vi "Get spectra Freq.vi"() -> (5 "Plug in titles":string[](array[string]), 7 "Plug in values":string[](array[string]))   [LabVIEW 2021]
uses:
  Globals/Meas_global.vi
panel:
  in  "Channel Indices for Spectra":i32[](array[numeric])=[0]
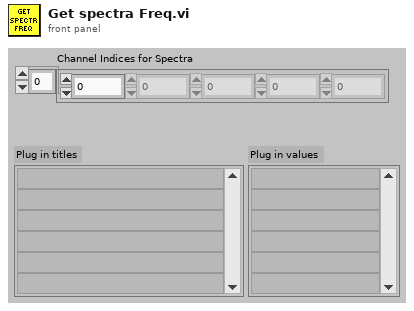
[diagram p1: front panel]
types:
  T1 = typedef "Setup.ctl" = enum16{"Run Program", "Show Setup", "Save Current Setup", "Setup Front Panel"}
  T2 = typedef "XY_Plot_Cluster.ctl" = cluster{"First Name":string, "Second Name":string, "X axis name":string, "Y axis name":string, "X array":dbl[], "Y array":dbl[], "Weighting":dbl[]}
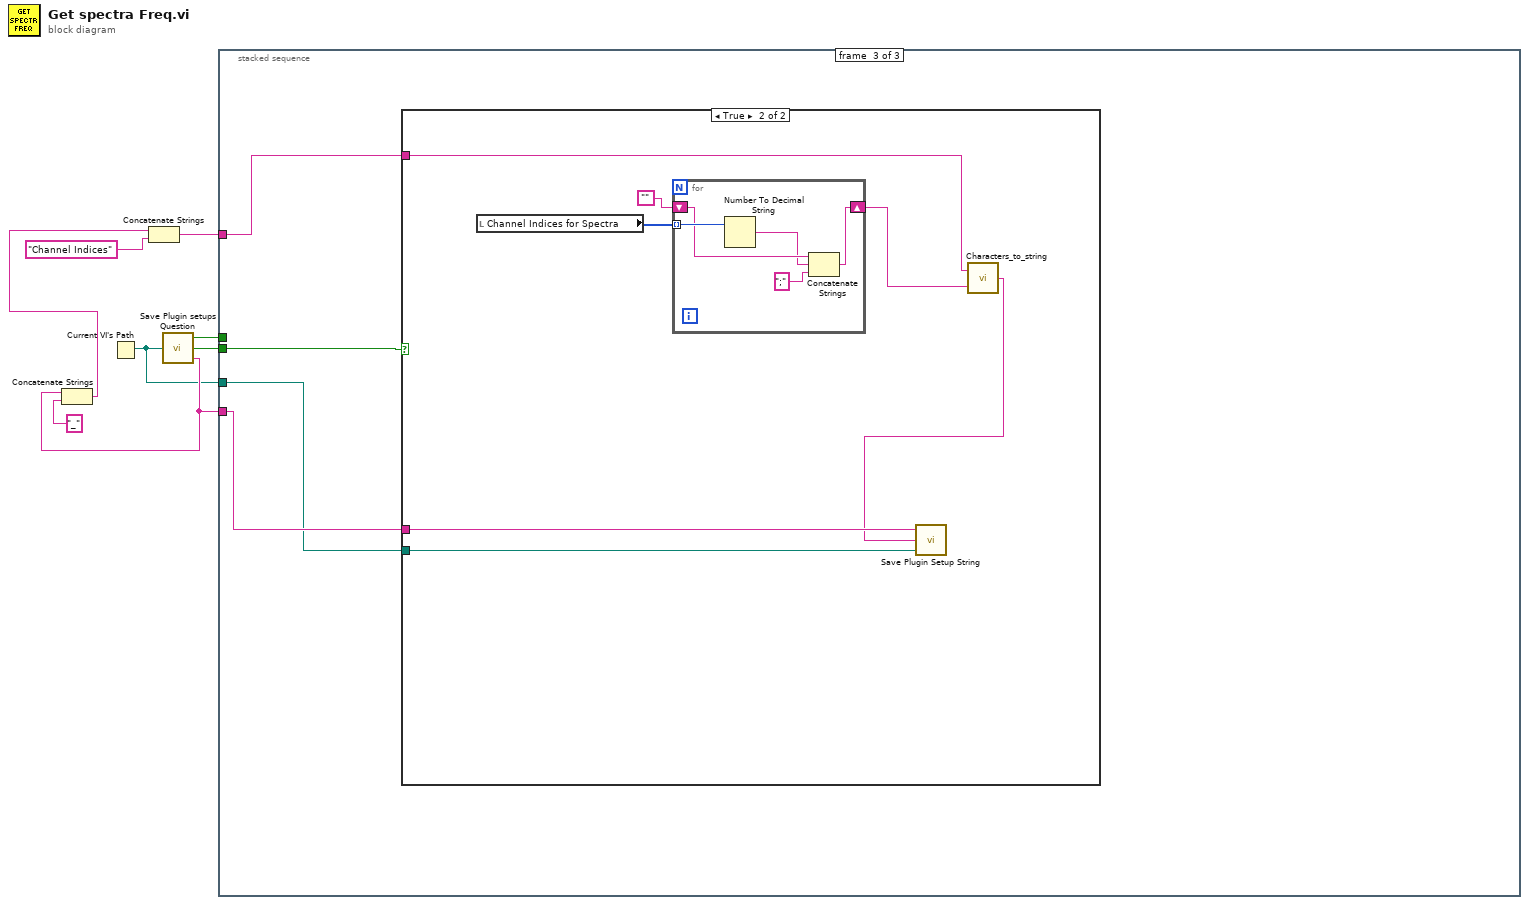
[diagram p0: block diagram]
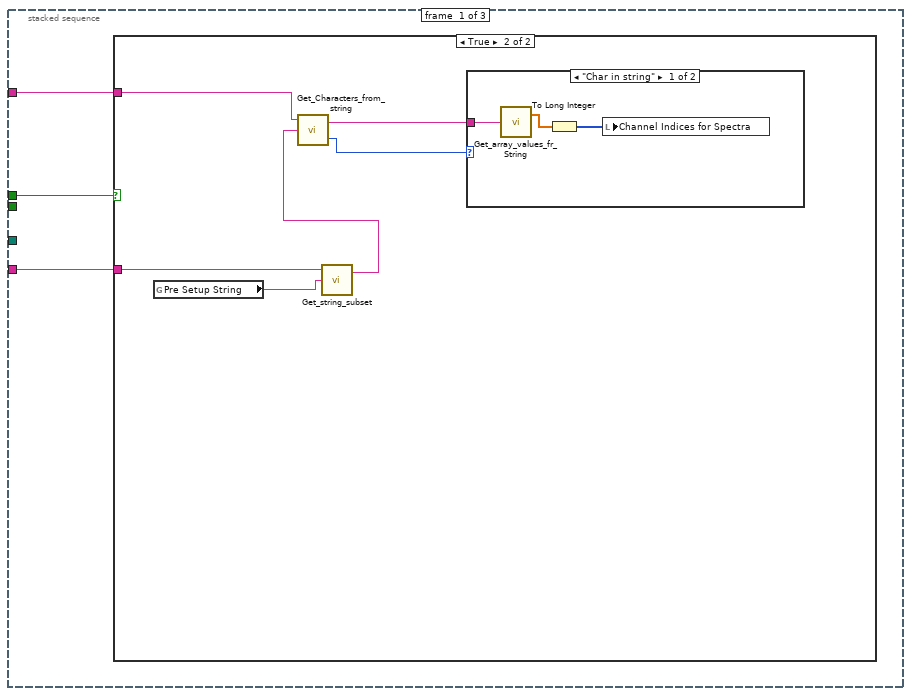
[diagram p2: hidden frame]
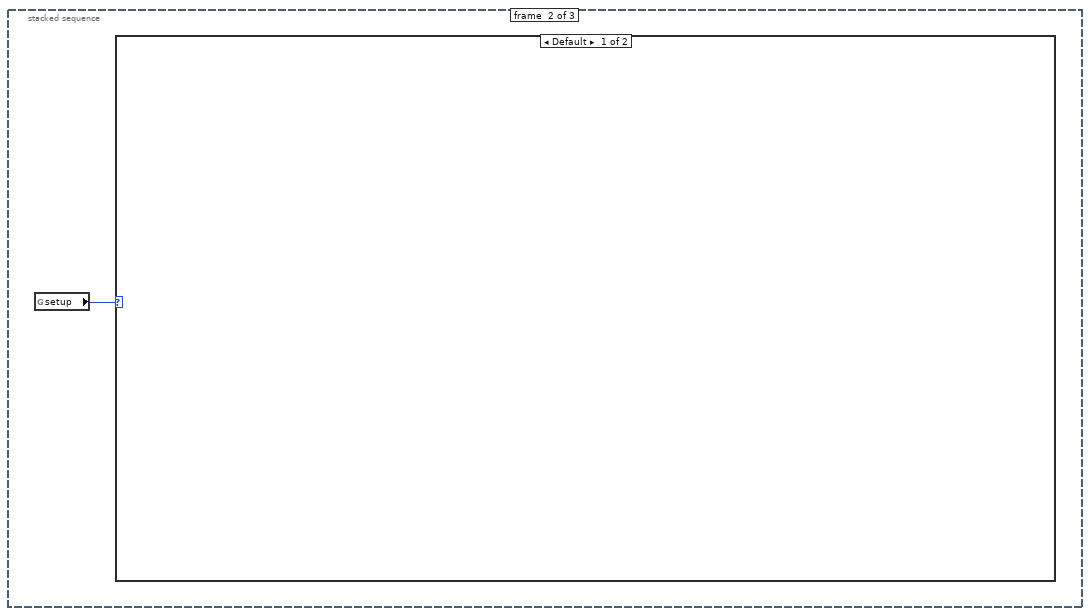
[diagram p5: hidden frame]
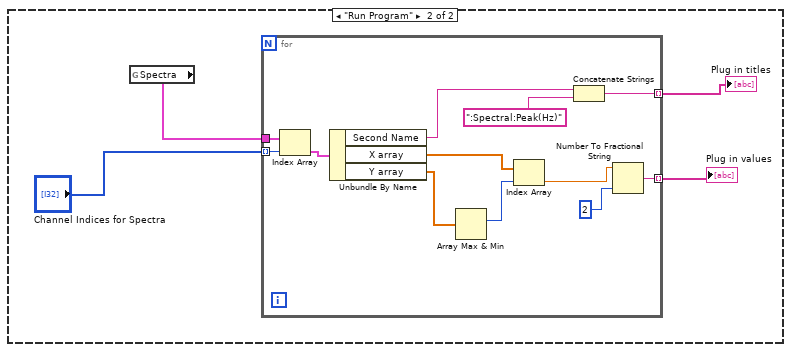
[diagram p6: hidden frame]
diagram:
  n1 = Current VI's Path() -> (path=w1:path)
  n2 = call "Save Plugin setups Question.vi"("VI path"=w1) -> ("Load Plugin Setup"=w8:bool, "Save Plugin Setup"=w2:bool, "Plugin_Label"=w3:string)
  n3 = Concatenate Strings(w3, "_" ("string")) -> (w5:string)
  n4 = Concatenate Strings(w5, "Channel Indices" ("Label for value")) -> (w4:string)
  n5 = stacked-sequence {
    tunnel: w8 -> [w11 _ _]
    tunnel: w4 -> [w10 _ w39]
    tunnel: w3 -> [w9 _ w40]
    tunnel: w2 -> [_ _ w41]
    tunnel: w1 -> [_ _ w38]
    frame #0 {
      n6 = case shown="True" w11 {
        tunnel: w10 -> [_ w17]
        tunnel: w9 -> [_ w14]
        frame False {
        }
        frame True {
          n7 = global read "Meas_global.vi" "Pre Setup String"() -> (w15:string)
          n8 = call "Get_string_subset.vi"("String to split"=w15, "File Label"=w14) -> ("Output string"=w13:string)  [unwired: 2 in, 1 out]
          n9 = call "Get_Characters_from_string.vi"("Input string"=w13, "Variable name"=w17) -> ("Status"=w12:enum16{"Char in string", "Char not in string"}, "Value"=w16:string)  [unwired: 1 in]
          n10 = case shown="\"Char in string\"" w12 {
            tunnel: w16 -> [w20 _]
            frame "Char in string" {
              n11 = call "Get_array_values_fr_String.vi"("String Value"=w20) -> ("Numeric Array"=w19:dbl[])  [unwired: 1 out]
              n12 = To Long Integer(number=w19) -> (32bit integer=w18:i32[])
              n13 = local write "Channel Indices for Spectra"(w18) -> ()
            }
            frame "Char not in string" {
            }
          }
        }
      }
    }
    frame #1 {
      n14 = global read "Meas_global.vi" "setup"() -> (w21:T1)
      n15 = case shown="Default" w21 {
        frame Default {
        }
        frame "Run Program" {
          n16 = global read "Meas_global.vi" "Spectra"() -> (w25:T2[])
          n17 = for {
            tunnel: w25 -> [w28]
            tunnel: [w32] -> w24 mode=indexing
            tunnel: [w29] -> w23 mode=indexing
            tunnel: "Channel Indices for Spectra" -> [w26] mode=indexing
            n18 = Index Array(array=w28, index=w26) -> (element=w27:T2)
            n19 = Unbundle By Name(w27) -> ("Second Name"=w34:string, "X array"=w36:dbl[], "Y array"=w37:dbl[])
            n20 = Array Max & Min(array=w37) -> (max index (indices)=w35:i32)  [unwired: 3 out]
            n21 = Index Array(array=w36, index=w35) -> (element=w31:dbl)
            n22 = Concatenate Strings(w34, ":Spectral:Peak(Hz)" ("string")) -> (w32:string)
            n23 = Number To Fractional String(number=w31, precision (6)=i16 2) -> (F-format string=w29:string)  [unwired: 2 in]
          }
          "Plug in titles" <- w24
          "Plug in values" <- w23
        }
      }
    }
    frame #2 {
      n24 = case shown="True" w41 {
        tunnel: w40 -> [_ w48]
        tunnel: w39 -> [_ w44]
        tunnel: w38 -> [_ w42]
        frame False {
        }
        frame True {
          n25 = local read "Channel Indices for Spectra"() -> (w47:i32[])
          n26 = for {
            tunnel: w47 -> [w53] mode=indexing
            shift-right: [w49] -> w45
            shift-left: "" -> [w52]
            n27 = Number To Decimal String(number=w53) -> (decimal integer string=w51:string)  [unwired: 1 in]
            n28 = Concatenate Strings(w52, w51, ";") -> (w49:string)
          }
          n29 = call "Characters_to_string.vi"("Characters to write"=w45, "Label for characters"=w44) -> ("Output string"=w43:string)  [unwired: 1 in]
          n30 = call "Save Plugin Setup String.vi"("Plug In Pathname"=w42, "Setup String to Save"=w43, "PlugIn Label"=w48) -> ()  [unwired: 2 in]
        }
      }
    }
  }
